vi "Piston Comp.vi"(6 "Abort":refnum<vi>, 7 "Step Size":dbl, 8 "Step #":i32, 9 "Original Position":dbl, 10 "Action":enum16{"MOVE", "BACK TO ORIGINE"}(ring)) -> (3 "position":dbl)   [LabVIEW 2014]
uses:
  Controls/StageStates.ctl
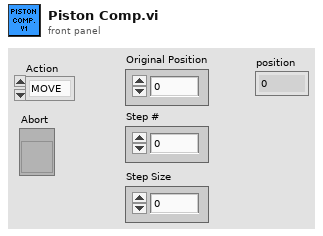
[diagram p1: front panel]
types:
  T1 = typedef "StageStates.ctl" = enum16{"POSITION", "MVR", "MOVE", "HALT", "ONTARGET", "ERROR", "EXIT", "HOME", "ZEROPOS", "NANOPOS", "QUIT", "ANALOG"}
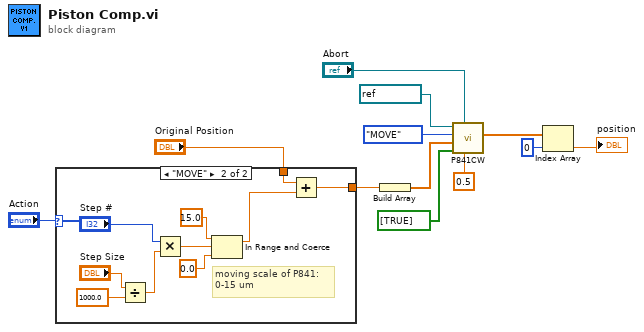
[diagram p0: block diagram]
diagram:
  n1 = case shown="\"MOVE\"" "Action" {
    tunnel: "Original Position" -> [w13 w22]
    tunnel: [w13 w21] -> w11
    frame "BACK TO ORIGINE" {
    }
    frame "MOVE" {
      # "moving scale of P841: \n0-15 um"
      n2 = Divide(x="Step Size", y=1000.0) -> (x/y=w18:dbl)
      n3 = Multiply(x="Step #", y=w18) -> (x*y=w17:dbl)
      n4 = In Range and Coerce(upper limit=15.0, x=w17, lower limit=0.0) -> (coerced(x)=w16:dbl)  [unwired: 1 out]
      n5 = Add(x=w22, y=w16) -> (x+y=w21:dbl)
    }
  }
  n6 = Build Array(w11) -> (w10:dbl[])
  n7 = call "P841CW.vi"("Velocity"=0.5, "Abort"="Abort", "Axis"=bool[] [TRUE], "Positions"=w10, "Action"=StageStates."MOVE", "VISA In"=refnum<visa-resource-name> "COM5" ("VISA resource name")) -> ("Position Out"=w3:dbl[])  [unwired: 2 in, 3 out]
  n8 = Index Array(array=w3, index=0) -> (element=→"position":dbl)
